vi "Set BufferLastReadingsDBL.vi"(10 "BufferLastReadings DBL":refnum<class "BufferLastReadings DBL.lvclass">, 11 "AI DAQmx Cont CFG in":refnum<class "AI DAQmx Cont CFG.lvclass">) -> (3 "AI DAQmx Cont CFG out":refnum<class "AI DAQmx Cont CFG.lvclass">)   [LabVIEW 2023, in "AI DAQmx Cont CFG.lvclass"]
uses:
  AI DAQmx Cont CFG.lvclass
  AI DAQmx Cont CFG.lvclass/AI DAQmx Cont CFG.ctl
  DAQmx/BufferLastReadingsDBL/BufferLastReadings DBL.lvclass
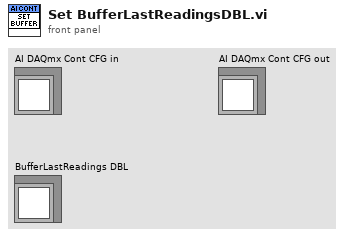
[diagram p1: front panel]
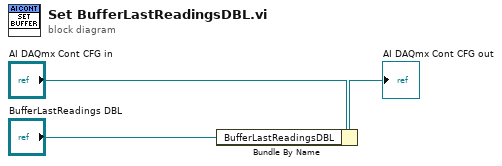
[diagram p0: block diagram]
diagram:
  n1 = Bundle By Name(cluster="AI DAQmx Cont CFG in", "BufferLastReadingsDBL"="BufferLastReadings DBL") -> (→"AI DAQmx Cont CFG out":refnum<class "AI DAQmx Cont CFG.lvclass">)
